vi "Velocity After Collision calcul.vi"(6 "v21":dbl, 7 "Alpha1 in":dbl, 8 "v12":dbl, 9 "u22":dbl, 10 "u11":dbl, 11 "Alpha2 in":dbl) -> (2 "V2 out":dbl[](array[numeric]), 3 "V1 out":dbl[](array[numeric]))   [LabVIEW 2021, in "Game Board.lvclass"]
doc: "MIT Licence\nCopyright (c) 2024 David Grollier"
uses:
  Game Board.lvclass
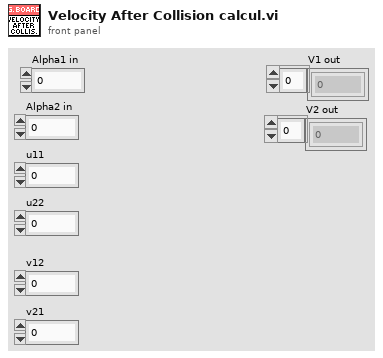
[diagram p1: front panel]
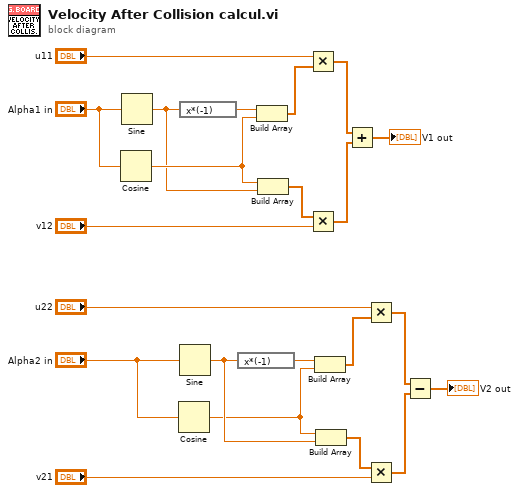
[diagram p0: block diagram]
diagram:
  n1 = Cosine(x="Alpha1 in") -> (cos(x)=w18:dbl)
  n2 = Sine(x="Alpha1 in") -> (sin(x)=w17:dbl)
  n3 = Cosine(x="Alpha2 in") -> (cos(x)=w7:dbl)
  n4 = expression code="x*(-1)"(w17) -> (w21:dbl)
  n5 = Sine(x="Alpha2 in") -> (sin(x)=w8:dbl)
  n6 = expression code="x*(-1)"(w8) -> (w5:dbl)
  n7 = Build Array(w21, w18) -> (w19:dbl[])
  n8 = Build Array(w18, w17) -> (w16:dbl[])
  n9 = Multiply(x="u11", y=w19) -> (x*y=w14:dbl[])
  n10 = Multiply(x=w16, y="v12") -> (x*y=w13:dbl[])
  n11 = Build Array(w5, w7) -> (w6:dbl[])
  n12 = Build Array(w7, w8) -> (w9:dbl[])
  n13 = Add(x=w14, y=w13) -> (x+y=→"V1 out":dbl[])
  n14 = Multiply(x="u22", y=w6) -> (x*y=w10:dbl[])
  n15 = Multiply(x=w9, y="v21") -> (x*y=w11:dbl[])
  n16 = Subtract(x=w10, y=w11) -> (x-y=→"V2 out":dbl[])
